vi "Get FIFO Usage.vi"(11 "FIFOusage":i32) -> (2 "function return":u32, 3 "FIFOusage out":i32)   [LabVIEW 2018, in "Copy of Andor SDK.lvlib"]
doc: "EXPNETTYPE unsigned int WINAPI GetFIFOUsage(int * FIFOusage);"
uses:
  Copy of Andor SDK.lvlib
  <userlib>/Andor SDK/ATMCD32D.dll
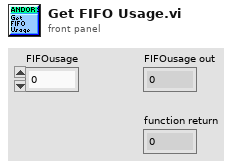
[diagram p1: front panel]
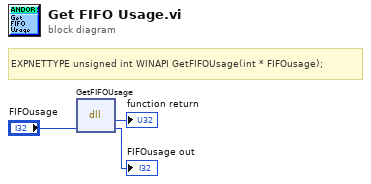
[diagram p0: block diagram]
diagram:
  # "EXPNETTYPE unsigned int WINAPI GetFIFOUsage(int * FIFOusage);"
  n1 = dll-call lib="C:/Program Files (x86)/National Instruments/LabVIEW 2018/user.lib/Andor SDK/ATMCD32D.*" fn="GetFIFOUsage"("FIFOusage"="FIFOusage") -> (→"function return":u32, "FIFOusage"=→"FIFOusage out":i32)  [unwired: 3 in, 2 out]
